vi "Check for valid PF.vi"(5 "Min V":dbl, 6 "Init":bool, 7 "Min I":dbl, 8 "PF In":dbl, 9 "VOLTS":dbl, 11 "Current":dbl) -> (0 "PF Out":dbl, 1 "V Out":dbl, 3 "I Out":dbl)   [LabVIEW 2017]
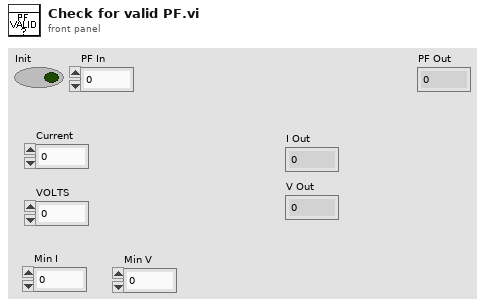
[diagram p1: front panel]
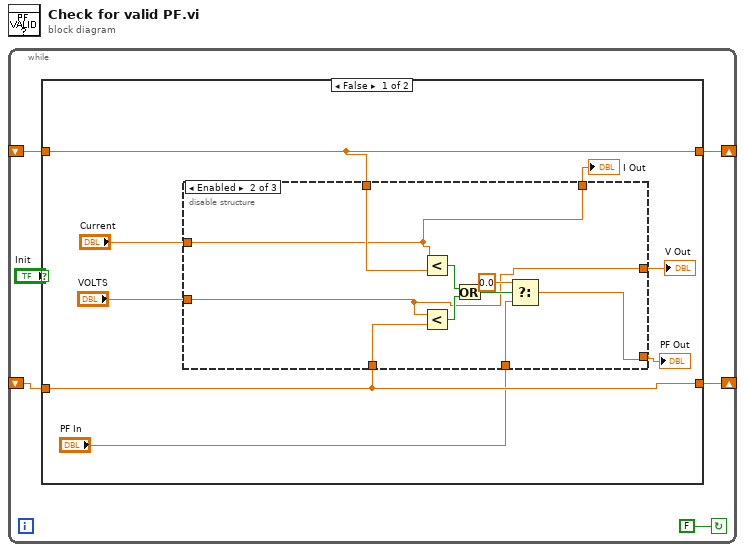
[diagram p0: block diagram]
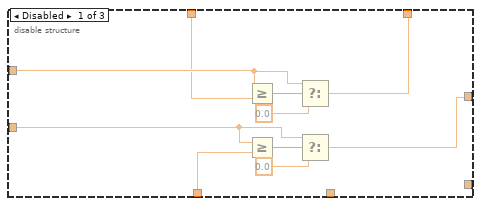
[diagram p2: hidden frame]
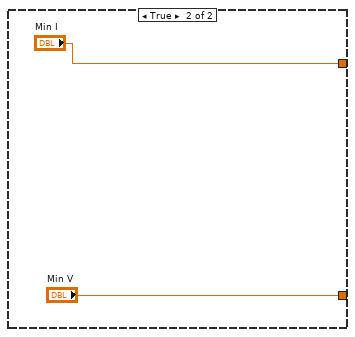
[diagram p4: hidden frame]
diagram:
  n1 = while {
    shift-right: [w3] -> _
    shift-left: _ -> [w2]
    shift-right: [w4] -> _
    shift-left: _ -> [w1]
    stop <- FALSE continue-if-true
    n2 = case shown="False" "Init" {
      tunnel: [w11 "Min V"] -> w4
      tunnel: [w12 "Min I"] -> w3
      tunnel: w2 -> [w12 _]
      tunnel: w1 -> [w11 _]
      frame False {
        n3 = disable-structure shown="Enabled" {
          disable-tunnel: "Current" -> [w20 w32 _]
          disable-tunnel: "VOLTS" -> [w19 w25 _]
          disable-tunnel: w12 -> [w18 w34 _]
          disable-tunnel: w11 -> [w17 w33 _]
          disable-tunnel: [w16 w32 _] -> w10
          disable-tunnel: [w15 w25 _] -> w9
          disable-tunnel: "PF In" -> [_ w28 _]
          disable-tunnel: [_ w27 _] -> w7
          frame Disabled {
            n4 = Greater Or Equal?(x=w20, y=w18) -> (x >= y?=w21:bool)
            n5 = Greater Or Equal?(x=w19, y=w17) -> (x >= y?=w24:bool)
            n6 = Select(t=w20, s=w21, f=0.0) -> (s? t:f=w16:dbl)
            n7 = Select(t=w19, s=w24, f=0.0) -> (s? t:f=w15:dbl)
          }
          frame Enabled {
            n8 = Less?(x=w32, y=w34) -> (x < y?=w30:bool)
            n9 = Less?(x=w25, y=w33) -> (x < y?=w31:bool)
            n10 = Or(x=w30, y=w31) -> (x .or. y?=w29:bool)
            n11 = Select(t=0.0, s=w29, f=w28) -> (s? t:f=w27:dbl)
          }
          frame Disabled {
          }
        }
        "I Out" <- w10
        "V Out" <- w9
        "PF Out" <- w7
      }
      frame True {
      }
    }
  }
